vi "Connect.vi"(0 "STOMP in":refnum<class "STOMP.lvclass">, 1 "address":string="localhost", 2 "port":u16=61613, 4 "timeout ms (60000)":i32=60000, 5 "error in":errorcluster) -> (14 "STOMP out":refnum<class "STOMP.lvclass">, 19 "error out":errorcluster)   [LabVIEW 2017, in "LabVIEW STOMP.lvlib" / "STOMP.lvclass"]
uses:
  STOMP.lvclass
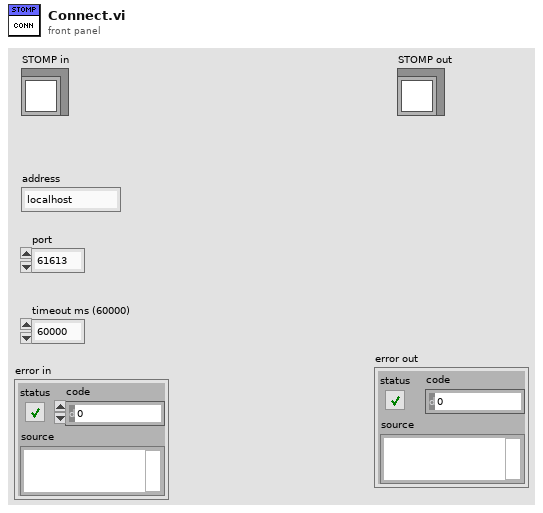
[diagram p1: front panel]
types:
  T1 = typedef "LabVIEW STOMP.lvlib/STOMP.lvclass/Type_ServerFrame.ctl" = cluster{"Type":T2, "Headers":cluster{"Header":string, "Value":string}[], "Body":string}
  T2 = typedef "LabVIEW STOMP.lvlib/STOMP.lvclass/Type_ServerFrameType.ctl" = enum16{"Undefined", "MESSAGE", "CONNECTED", "RECEIPT", "ERROR"}
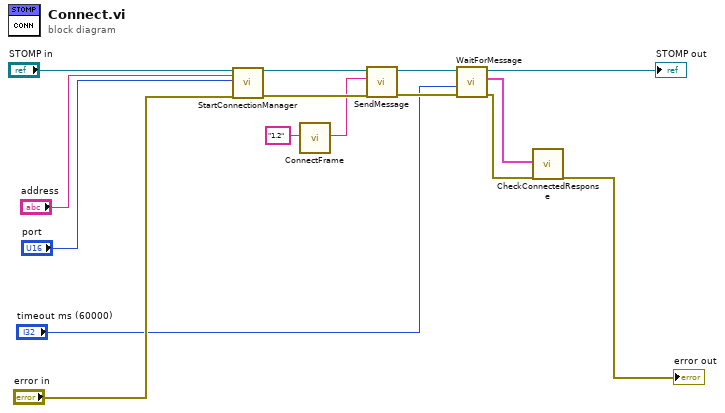
[diagram p0: block diagram]
diagram:
  n1 = call-dynamic "StartConnectionManager.vi"("STOMP in"="STOMP in", "address"="address", "port"="port", "error in (no error)"="error in") -> ("STOMP out"=w14:refnum<class "STOMP.lvclass">, "error out"=w15:errorcluster)  [unwired: 14 in]
  n2 = call "ConnectFrame.vi"("version"="1.2") -> ("Connect Frame"=w13:string)  [unwired: 18 in]
  n3 = call-dynamic "SendMessage.vi"("error in (no error)"=w15, "data in"=w13, "STOMP in"=w14) -> ("error out"=w6:errorcluster, "STOMP out"=w7:refnum<class "STOMP.lvclass">)  [unwired: 7 in]
  n4 = call-dynamic "WaitForMessage.vi"("error in (no error)"=w6, "timeout in ms (10000)"="timeout ms (60000)", "STOMP in"=w7) -> ("error out"=w2:errorcluster, "message"=w3:T1, "STOMP out"=→"STOMP out":refnum<class "STOMP.lvclass">)  [unwired: 5 in, 1 out]
  n5 = call "CheckConnectedResponse.vi"("message"=w3, "error in (no error)"=w2) -> ("error out"=→"error out":errorcluster)  [unwired: 17 in]
